vi "All stations Seq Set.vi"(10 "all state configs":T1[](array[typedef])) -> ()   [LabVIEW 2018]
uses:
  Crl defs/DataStream.ctl
  Crl defs/one state paths config.ctl
  Crl defs/one state prints config.ctl
  Communication connection/Crl defs/print config.ctl
  Crl defs/one state scans config.ctl
  Communication connection/Crl defs/scanner config.ctl
  Crl defs/one state tags config.ctl
  Crl defs/PLC_bool tags.ctl
  DataSocket/Crl defs/DataSocket_Tags.ctl
  Crl defs/PLC_real tags.ctl
  Crl defs/PLC_string tags.ctl
  Crl defs/one state msic config.ctl
  Sequence/type defs/Sequence Info.ctl
  Crl defs/one state power supply config.ctl
  Crl defs/motor operating data.ctl
  Crl defs/one state screw config.ctl
  Crl defs/xls.data'S buffer.ctl
  Crl defs/XLS.header configs.ctl
panel:
  in  "SunshadeCode and Color":bool
  in  "Part Type":u16(ring) items=["V61", "B16", "CC02"]
  in  "Button 20":bool
  in  "Button 19":bool
  in  "Button 18":bool
  in  "Button 17":bool
  in  "Exit":bool
  in  "Button 16":bool
  in  "Button 15":bool
  in  "Button 14":bool
  in  "Button 13":bool
  in  "Button 12":bool
  in  "Button 11":bool
  in  "Button 10":bool
  in  "Button 9":bool
  in  "Button 8":bool
  in  "Button 7":bool
  in  "Button 6":bool
  in  "Button 5":bool
  in  "Button 4":bool
  in  "Button 3":bool
  in  "Button 2":bool
  in  "Button 1":bool
  # "All Type Test Sequence"
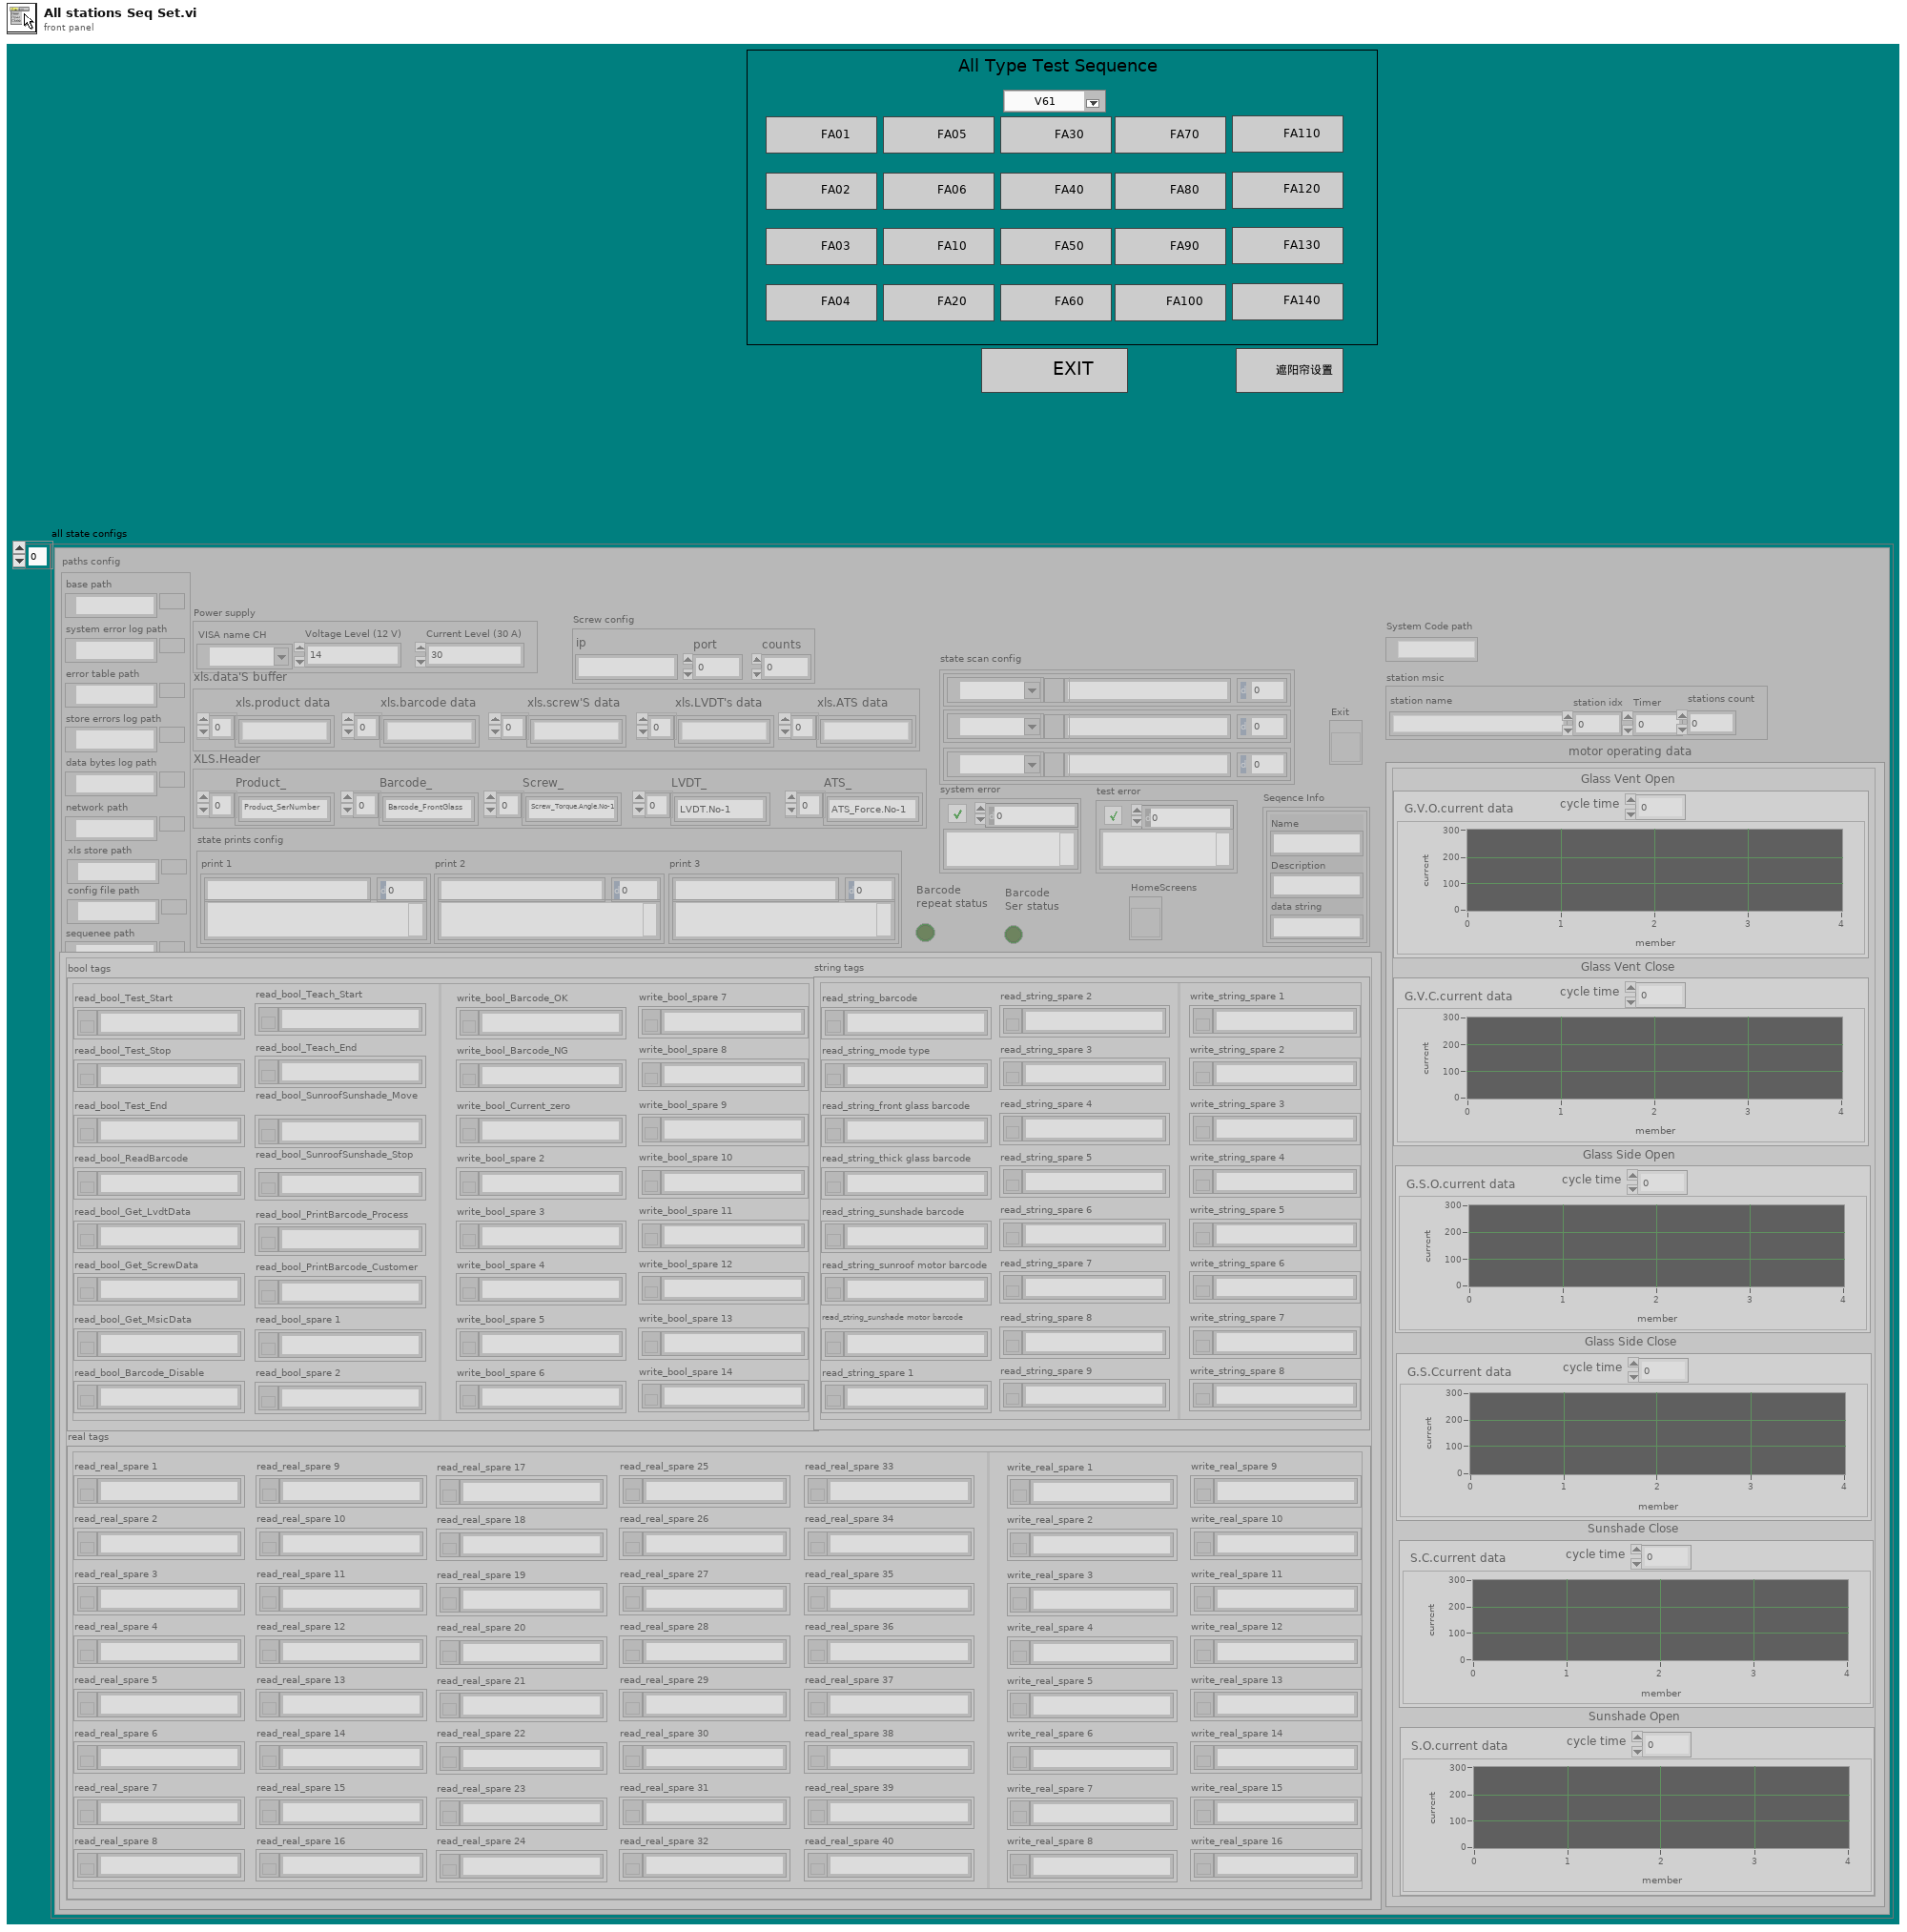
[diagram p1: front panel]
types:
  T1 = typedef "DataStream.ctl" = cluster{"paths config":T2, "state prints config":T3, "state scan config":T5, "all tags of plc":T7, "station msic":T12, "test error":errorcluster, "system error":errorcluster, "Seqence Info":T13[], "Power supply":T14, "motor operating data":T15, "Screw config":T16, "xls.data'S buffer":T17, "XLS.Header":T18, "Barcode\nrepeat status":bool, "Barcode\nSer status":bool, "System Code path":path, "Exit":refnum<vi>, "HomeScreens":refnum<vi>}
  T2 = typedef "one state paths config.ctl" = cluster{"base path":path, "system error log path":path, "error table path":path, "store errors log path":path, "data bytes log path":path, "network path":path, "xls store path":path, "config file path":path, "sequenee path":path}
  T3 = typedef "one state prints config.ctl" = cluster{"print 1":T4, "print 2":T4, "print 3":T4}
  T4 = typedef "print config.ctl" = cluster{"connect ip or coms":string, "port":u16, "print strings":string}
  T5 = typedef "one state scans config.ctl" = cluster{"scan 1 ":T6, "scan 2":T6, "scan 3":T6}
  T6 = typedef "scanner config.ctl" = cluster{"connect ip or coms":string, "port":u16, "tcp connect id":refnum<k5>, "VISA resource name":refnum<visa-resource-name>}
  T7 = typedef "one state tags config.ctl" = cluster{"bool tags":T8, "real tags":T10, "string tags":T11}
  T8 = typedef "PLC_bool tags.ctl" = cluster{"read_bool_Test_Start":T9, "read_bool_Test_Stop":T9, "read_bool_Test_End":T9, "read_bool_ReadBarcode":T9, "read_bool_Get_LvdtData":T9, "read_bool_Get_ScrewData":T9, "read_bool_Get_MsicData":T9, "read_bool_Barcode_Disable":T9, "read_bool_Teach_Start":T9, "read_bool_Teach_End":T9, "read_bool_SunroofSunshade_Move":T9, "read_bool_SunroofSunshade_Stop":T9, "read_bool_PrintBarcode_Process":T9, "read_bool_PrintBarcode_Customer":T9, "read_bool_spare 1":T9, "read_bool_spare 2":T9, "write_bool_Barcode_OK":T9, "write_bool_Barcode_NG":T9, "write_bool_Current_zero":T9, "write_bool_spare 2":T9, "write_bool_spare 3":T9, "write_bool_spare 4":T9, "write_bool_spare 5":T9, "write_bool_spare 6":T9, "write_bool_spare 7":T9, "write_bool_spare 8":T9, "write_bool_spare 9":T9, "write_bool_spare 10":T9, "write_bool_spare 11":T9, "write_bool_spare 12":T9, "write_bool_spare 13":T9, "write_bool_spare 14":T9}
  T9 = typedef "DataSocket_Tags.ctl" = cluster{"Ds ID":refnum<k13>, "Tag":string}
  T10 = typedef "PLC_real tags.ctl" = cluster{"read_real_spare 1":T9, "read_real_spare 2":T9, "read_real_spare 3":T9, "read_real_spare 4":T9, "read_real_spare 5":T9, "read_real_spare 6":T9, "read_real_spare 7":T9, "read_real_spare 8":T9, "read_real_spare 9":T9, "read_real_spare 10":T9, "read_real_spare 11":T9, "read_real_spare 12":T9, "read_real_spare 13":T9, "read_real_spare 14":T9, "read_real_spare 15":T9, "read_real_spare 16":T9, "read_real_spare 17":T9, "read_real_spare 18":T9, "read_real_spare 19":T9, "read_real_spare 20":T9, "read_real_spare 21":T9, "read_real_spare 22":T9, "read_real_spare 23":T9, "read_real_spare 24":T9, "read_real_spare 25":T9, "read_real_spare 26":T9, "read_real_spare 27":T9, "read_real_spare 28":T9, "read_real_spare 29":T9, "read_real_spare 30":T9, "read_real_spare 31":T9, "read_real_spare 32":T9, "read_real_spare 33":T9, "read_real_spare 34":T9, "read_real_spare 35":T9, "read_real_spare 36":T9, "read_real_spare 37":T9, "read_real_spare 38":T9, "read_real_spare 39":T9, "read_real_spare 40":T9, "write_real_spare 1":T9, "write_real_spare 2":T9, "write_real_spare 3":T9, "write_real_spare 4":T9, "write_real_spare 5":T9, "write_real_spare 6":T9, "write_real_spare 7":T9, "write_real_spare 8":T9, "write_real_spare 9":T9, "write_real_spare 10":T9, "write_real_spare 11":T9, "write_real_spare 12":T9, "write_real_spare 13":T9, "write_real_spare 14":T9, "write_real_spare 15":T9, "write_real_spare 16":T9}
  T11 = typedef "PLC_string tags.ctl" = cluster{"read_string_barcode":T9, "read_string_mode type":T9, "read_string_front glass barcode":T9, "read_string_thick glass barcode":T9, "read_string_sunshade barcode":T9, "read_string_sunroof motor barcode":T9, "read_string_sunshade motor barcode\n":T9, "read_string_spare 1":T9, "read_string_spare 2":T9, "read_string_spare 3":T9, "read_string_spare 4":T9, "read_string_spare 5":T9, "read_string_spare 6":T9, "read_string_spare 7":T9, "read_string_spare 8":T9, "read_string_spare 9":T9, "write_string_spare 1":T9, "write_string_spare 2":T9, "write_string_spare 3":T9, "write_string_spare 4":T9, "write_string_spare 5":T9, "write_string_spare 6":T9, "write_string_spare 7":T9, "write_string_spare 8":T9}
  T12 = typedef "one state msic config.ctl" = cluster{"station name":string, "Timer":u32, "station idx":i32, "stations count":i32}
  T13 = typedef "Sequence Info.ctl" = cluster{"Name":string, "Description":string, "data string":string}
  T14 = typedef "one state power supply config.ctl" = cluster{"VISA name CH":refnum<visa-resource-name>, "Voltage Level (12 V)":dbl, "Current Level (30 A)":dbl}
  T15 = typedef "motor operating data.ctl" = cluster{"Glass Vent Open":cluster{"cycle time":sgl, "G.V.O.current data":sgl[]}, "Glass Vent Close":cluster{"cycle time":sgl, "G.V.C.current data":sgl[]}, "Glass Side Open":cluster{"cycle time":sgl, "G.S.O.current data":sgl[]}, "Glass Side Close":cluster{"cycle time":sgl, "G.S.Ccurrent data":sgl[]}, "Sunshade Close":cluster{"cycle time":sgl, "S.C.current data":sgl[]}, "Sunshade Open":cluster{"cycle time":sgl, "S.O.current data":sgl[]}}
  T16 = typedef "one state screw config.ctl" = cluster{"ip":string, "port":u16, "counts":u16}
  T17 = typedef "xls.data'S buffer.ctl" = cluster{"xls.product data":string[], "xls.barcode data":string[], "xls.screw'S data":string[], "xls.LVDT's data":string[], "xls.ATS data":string[]}
  T18 = typedef "XLS.header configs.ctl" = cluster{"Product_":string[], "Barcode_":string[], "Screw_":string[], "LVDT_":string[], "ATS_":string[]}
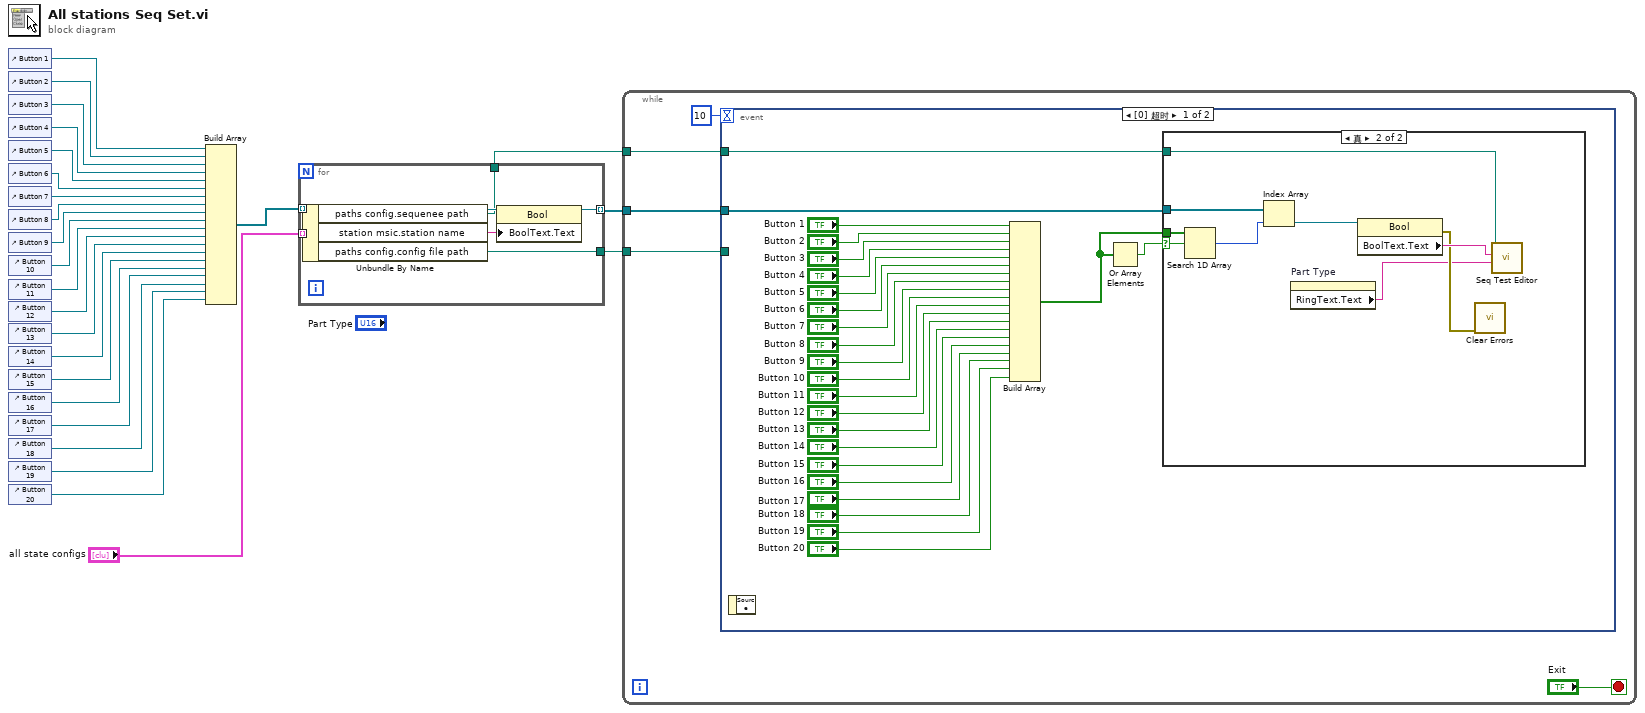
[diagram p0: block diagram]
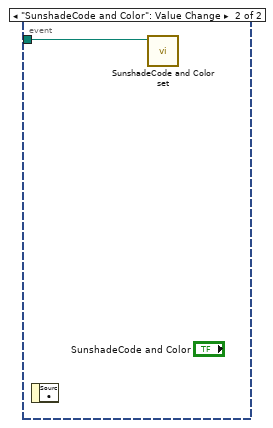
[diagram p3: hidden frame]
diagram:
  n1 = control-ref of="Button 1"() -> (w25:refnum<vi>)
  n2 = control-ref of="Button 2"() -> (w24:refnum<vi>)
  n3 = control-ref of="Button 3"() -> (w23:refnum<vi>)
  n4 = control-ref of="Button 4"() -> (w22:refnum<vi>)
  n5 = control-ref of="Button 5"() -> (w21:refnum<vi>)
  n6 = control-ref of="Button 6"() -> (w20:refnum<vi>)
  n7 = control-ref of="Button 7"() -> (w19:refnum<vi>)
  n8 = control-ref of="Button 8"() -> (w18:refnum<vi>)
  n9 = control-ref of="Button 9"() -> (w17:refnum<vi>)
  n10 = control-ref of="Button 10"() -> (w16:refnum<vi>)
  n11 = control-ref of="Button 11"() -> (w15:refnum<vi>)
  n12 = control-ref of="Button 12"() -> (w14:refnum<vi>)
  n13 = control-ref of="Button 13"() -> (w13:refnum<vi>)
  n14 = control-ref of="Button 14"() -> (w12:refnum<vi>)
  n15 = control-ref of="Button 15"() -> (w11:refnum<vi>)
  n16 = control-ref of="Button 16"() -> (w10:refnum<vi>)
  n17 = control-ref of="Button 17"() -> (w6:refnum<vi>)
  n18 = control-ref of="Button 18"() -> (w5:refnum<vi>)
  n19 = control-ref of="Button 19"() -> (w4:refnum<vi>)
  n20 = control-ref of="Button 20"() -> (w3:refnum<vi>)
  n21 = Build Array(w25, w24, w23, w22, w21, w20, w19, w18, w17, w16, w15, w14, w13, w12, w11, w10, w6, w5, w4, w3) -> (w9:refnum<vi>[])
  n22 = for {
    tunnel: w9 -> [w31] mode=indexing
    tunnel: "all state configs" -> [w30] mode=indexing
    tunnel: [w28] -> w7 mode=indexing
    tunnel: [w27] -> w2
    tunnel: [w26] -> w1
    n23 = Unbundle By Name(w30) -> ("paths config.sequenee path"=w26:path, "station msic.station name"=w29:string, "paths config.config file path"=w27:path)
    n24 = property class="Bool"(reference=w31, "BoolText.Text"=w29) -> (reference out=w28:refnum<vi>)  [unwired: 1 in, 1 out]
  }
  n25 = while {
    tunnel: w7 -> [w35]
    tunnel: w1 -> [w33]
    tunnel: w2 -> [w32]
    stop <- "Exit" stop-if-true
    n26 = event shown="[0] 超时" {
      selector: _ -> [_ _]
      dyn-events: _ -> [_ _]
      timeout: 10 -> [_ _]
      tunnel: w35 -> [w43 _]
      tunnel: w33 -> [w37 _]
      tunnel: w32 -> [_ w70]
      event Timeout {
        n27 = event-data() -> ()  [unwired: 1 in, 1 out]
        n28 = Build Array("Button 1", "Button 2", "Button 3", "Button 4", "Button 5", "Button 6", "Button 7", "Button 8", "Button 9", "Button 10", "Button 11", "Button 12", "Button 13", "Button 14", "Button 15", "Button 16", "Button 17", "Button 18", "Button 19", "Button 20") -> (w42:bool[])
        n29 = Or Array Elements(Boolean array=w42) -> (logical OR=w60:bool)
        n30 = case shown="真" w60 {
          selector: w60 -> [_ w65]
          tunnel: w42 -> [_ w69]
          tunnel: w43 -> [_ w68]
          tunnel: w37 -> [_ w61]
          frame False {
          }
          frame True {
            n31 = Search 1D Array(1D array=w69, element=w65) -> (index of element=w67:i32)  [unwired: 1 in]
            n32 = Index Array(array=w68, index=w67) -> (element=w66:refnum<vi>)
            n33 = property on="Part Type" class="Ring (严格)"() -> ("RingText.Text"=w62:string)  [unwired: 2 in, 2 out]
            n34 = property class="Bool"(reference=w66) -> (error out=w63:errorcluster, "BoolText.Text"=w64:string)  [unwired: 1 in, 1 out]
            n35 = call <vilib>:"Clear Errors.vi"("error in (no error)"=w63) -> ()  [unwired: 5 in, 2 out]
            n36 = call "Seq Test Editor.vi"("Part Type"=w62, "Station"=w64, "Base Path"=w61) -> ()  [unwired: 8 in, 1 out]
          }
        }
      }
      event "SunshadeCode and Color": Value Change {
        n37 = event-data() -> ()  [unwired: 1 in, 1 out]
        n38 = call "SunshadeCode and Color set.vi"("file path (dialog if empty)"=w70) -> ()  [unwired: 11 in]
      }
    }
  }
